vi "OpenTestFile.vi"(8 "ErrorArray In":errorcluster[](array[cluster])) -> (0 "ErrorArray Out":errorcluster[](array[cluster]), 1 "BusData":T2[](array[typedef]) {"clConfigOptions"."PHUNIT" max=16777216 step=1 format="%08d"; "clConfigOptions"."IDCODE" format="%02x"; "clConfigOptions"."TIME_BASE" max=16777216 step=1 format="%08d"; "ImpairReportArray"."Synx" format="%#_4g"; "EvtReportArray"."Synx" format="%#_4g"; "EvtConfig"."Reporting Rate" items=["10 FPS"=10, "12 FPS"=12, "15 FPS"=15, "20 FPS"=20, "25 FPS"=25, "30 FPS"=30, "50 FPS"=50, "60 FPS"=60]; "EvtConfig"."Nominal Frequency" items=["50 Hz"=50, "60 Hz"=60]}, 3 "TestFileRef out":T1)   [LabVIEW 2017, in "Framework.lvlib"]
uses:
  Framework.lvlib
  Bus_class/Public/TypeDefs/clBusData.ctl
  FrontPanel/TypeDefs/clEventConfig.ctl
  Modules/PmuImpairPlugins/PmuImpairPluginBase_class/TypeDefs/clImpairConfig.ctl
  Modules/EventPlugins/EventPluginBaseClass/TypeDefs/clEvtReportArray.ctl
  Modules/EventPlugins/EventPluginBaseClass/TypeDefs/clEvtReport.ctl
  Modules/EventPlugins/EventPluginBaseClass/TypeDefs/dblEvtSignalArray.ctl
  Modules/NetworkImpairmentModule/PublicAPI/Arguments/Broadcasts/dblNetworkTime.ctl
  Modules/NetworkImpairmentModule/PublicAPI/Arguments/Broadcasts/dblPktLoss.ctl
  Modules/FlagImpairModule/PublicAPI/Arguments/Broadcasts/ui32FlagImpairmentArray.ctl
  Modules/OutputToFilePlugins/OutputToFileBasePlugin/Typedefs/PmuCfgOpt.ctl
  <vilib>/Utility/config.llb/Config Data RefNum.ctl
  Bus_class/Bus.lvclass
  Modules/EventPlugins/EventPluginBaseClass/EventPluginBaseClass.lvclass
  Modules/NetworkImpairmentModule/NetworkImpairmentModule.lvlib
  Modules/FlagImpairModule/FlagImpairModule.lvlib
  Modules/OutputToFilePlugins/OutputToFileBasePlugin/OutputToFileBasePlugin.lvclass
  Modules/PmuImpairPlugins/PmuImpairPluginBase_class/PmuImpairPluginBase.lvclass
  <vilib>/Utility/config.llb/NI_LVConfig.lvlib
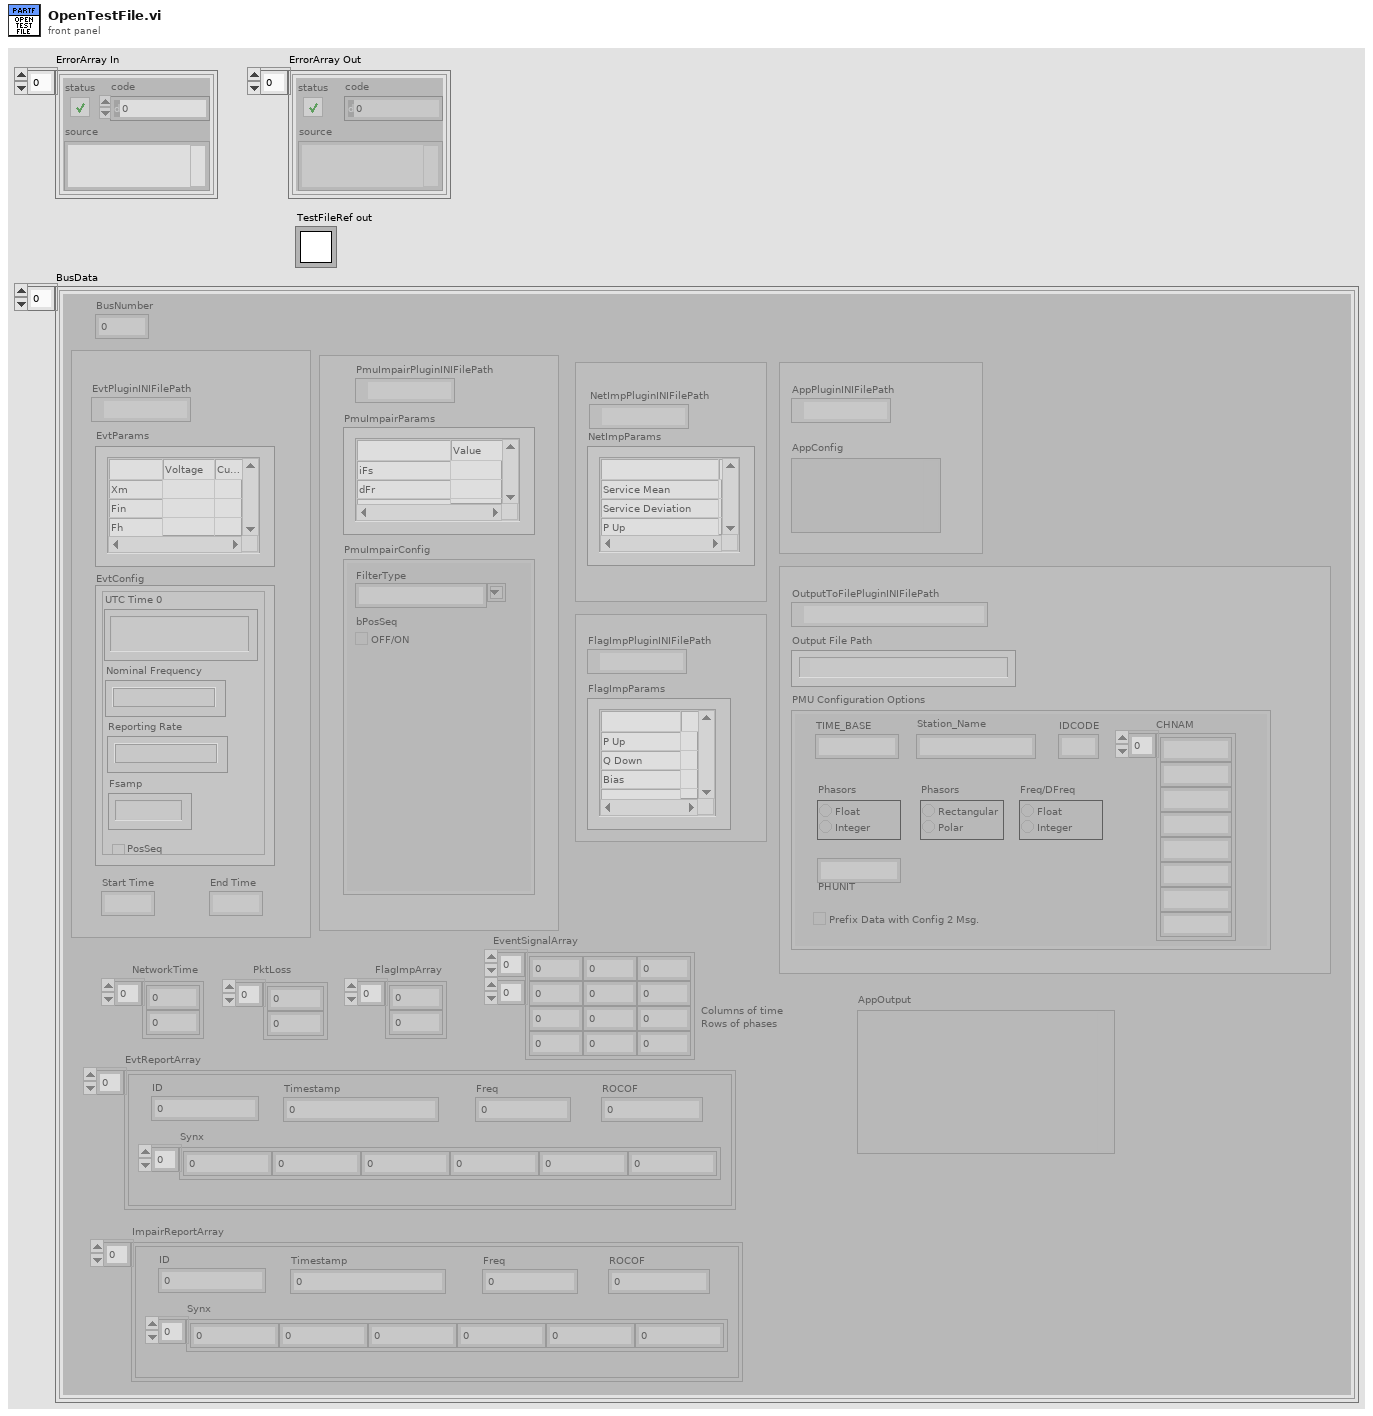
[diagram p1: front panel]
types:
  T1 = typedef "NI_LVConfig.lvlib/Config Data RefNum.ctl" = refnum<k1>
  T2 = typedef "Bus_class.lvlib/Bus.lvclass/clBusData.ctl" = cluster{"BusNumber":u8, "EvtPluginINIFilePath":path, "EvtParams":string[][], "EvtConfig":T3, "Start Time":dbl, "End Time":dbl, "PmuImpairPluginINIFilePath":path, "PmuImpairParams ":string[][], "PmuImpairConfig":T4, "NetImpPluginINIFilePath":path, "NetImpParams":string[][], "FlagImpPluginINIFilePath":path, "FlagImpParams":string[][], "EvtReportArray":T5, "EventSignalArray":T7, "ImpairReportArray":T5, "NetworkTime":T8, "PktLoss":T9, "FlagImpArray":T10, "OutputToFilePluginINIFilePath":path, "Output File Path":path, "clConfigOptions":T11, "AppPluginINIFilePath":path, "AppConfig":variant, "AppOutput":variant}
  T3 = typedef "Framework.lvlib/clEventConfig.ctl" = cluster{"UTC Time 0":timestamp, "Nominal Frequency":u16, "Reporting Rate":u16, "Fsamp":u32, "PosSeq":bool}
  T4 = typedef "PmuImpairPlugins.lvlib/PmuImpairPluginBase.lvclass/clImpairConfig.ctl" = cluster{"FilterType":string, "bPosSeq":bool}
  T5 = typedef "EventPlugins.lvlib/EventPluginBaseClass.lvclass/clEvtReportArray.ctl" = T6[]
  T6 = typedef "EventPlugins.lvlib/EventPluginBaseClass.lvclass/clEvtReport.ctl" = cluster{"Timestamp":dbl, "Synx":cdb[], "Freq":dbl, "ROCOF":dbl, "ID":i16}
  T7 = typedef "EventPlugins.lvlib/EventPluginBaseClass.lvclass/dblEvtSignalArray.ctl" = dbl[][]
  T8 = typedef "NetworkImpairmentModule.lvlib/dblNetworkTime.ctl" = dbl[]
  T9 = typedef "NetworkImpairmentModule.lvlib/dblPktLoss.ctl" = dbl[]
  T10 = typedef "FlagImpairModule.lvlib/ui32FlagImpairmentArray.ctl" = u32[]
  T11 = typedef "OutputToFilePlugins.lvlib/OutputToFileBasePlugin.lvclass/PmuCfgOpt.ctl" = cluster{"TIME_BASE":u64, "STN":string, "IDCODE":u16, "rdoPolRect":enum32{"Rectangular", "Polar"}, "rdoFloatInt":enum32{"Float", "Integer"}, "PHUNIT":u64, "rdoFreqDfreq":enum32{"Float", "Integer"}, "CHNAM":string[], "chkCfg2Prefix":bool}
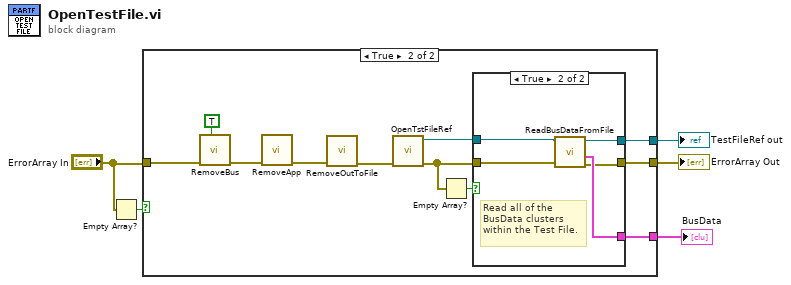
[diagram p0: block diagram]
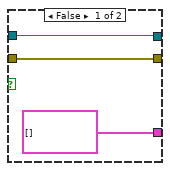
[diagram p3: hidden frame]
diagram:
  n1 = Empty Array?(array="ErrorArray In") -> (empty?=w5:bool)
  n2 = case shown="True" w5 {
    tunnel: "ErrorArray In" -> [w7 w18]
    tunnel: [w7 w10] -> w4
    tunnel: [T2[] [] ("BusData") w16] -> w3
    tunnel: [_ w8] -> w1
    frame False {
    }
    frame True {
      n3 = call "RemoveBus.vi"("Remove All? (F)"=TRUE ("Remove All?"), "ErrorArray In"=w18) -> ("ErrorArray Out"=w15:errorcluster[])  [unwired: 9 in]
      n4 = call "RemoveApp.vi"("ErrorArray In"=w15) -> ("ErrorArray Out"=w14:errorcluster[])  [unwired: 10 in]
      n5 = call "RemoveOutToFile.vi"("ErrorArray In"=w14) -> ("ErrorArray Out"=w13:errorcluster[])  [unwired: 10 in]
      n6 = call "OpenTstFileRef.vi"("ErrorArray"=w13) -> ("ErrorArray"=w11:errorcluster[], "refnum"=w9:T1)  [unwired: 9 in]
      n7 = Empty Array?(array=w11) -> (empty?=w12:bool)
      n8 = case shown="True" w12 {
        tunnel: [w21 w22] -> w10
        tunnel: w11 -> [w21 w26]
        tunnel: [T2[] [] ("BusData") w25] -> w16
        tunnel: w9 -> [w19 w24]
        tunnel: [w19 w23] -> w8
        frame False {
        }
        frame True {
          # "Read all of the\nBusData clusters\nwithin the Test File."
          n9 = call "ReadBusDataFromFile.vi"("ErrorArray In"=w26, "TestFileRef In"=w24) -> ("ErrorArray Out"=w22:errorcluster[], "BusData"=w25:T2[], "refnum out"=w23:T1)  [unwired: 7 in]
        }
      }
    }
  }
  "ErrorArray Out" <- w4
  "BusData" <- w3
  "TestFileRef out" <- w1
